vi "microstepping.vi"(4 "1 per 8 step":bool, 5 "1 per 16 step":bool, 6 "1 per 2 step":bool, 7 "full step":bool, 8 "1 per 4 step":bool, 9 "radius":dbl=5.0, 10 "arcLength":dbl=10.0, 11 "task/channels in microstepping":refnum<k21>) -> (0 "number of samples written":u32, 3 "convertedTodegree":dbl)   [LabVIEW 2016]
uses:
  <vilib>/DAQmx/write.llb/DAQmx Write (Digital 1D Bool NChan 1Samp 1Line).vi
  <vilib>/DAQmx/miscellaneous.llb/DAQmx Fill In Error Info.vi
panel:
  out "Numeric":i32
  out "full":dbl
  out "1 per 16":dbl
  in  "task/channels in trotate orientation":refnum<k21>="orientationPort2"
  in  "task/channels in toggle (step)":refnum<k21>="port01enable"
  in  "rotate orientation":string(combo)="clockwise"
  in  "steeper Motor Speed":u32(knob) scale=10.0..100.0
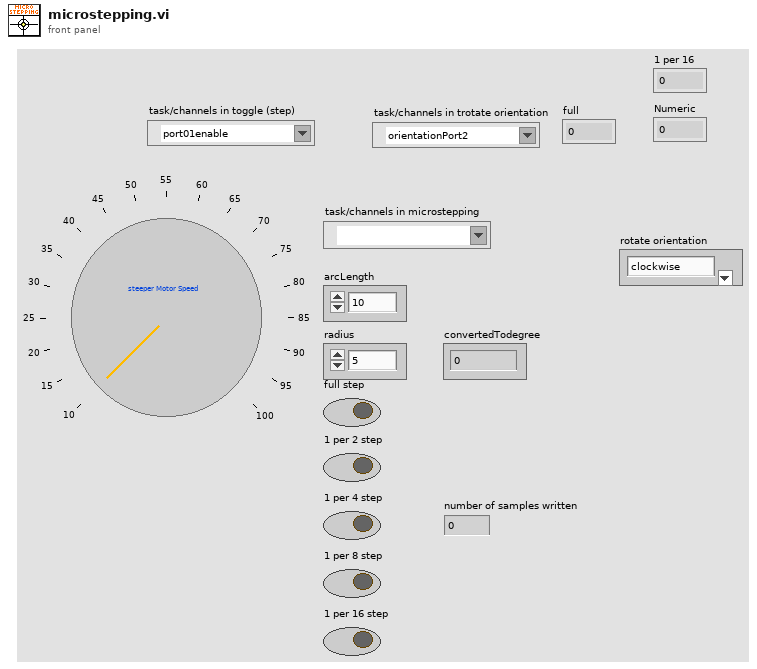
[diagram p1: front panel]
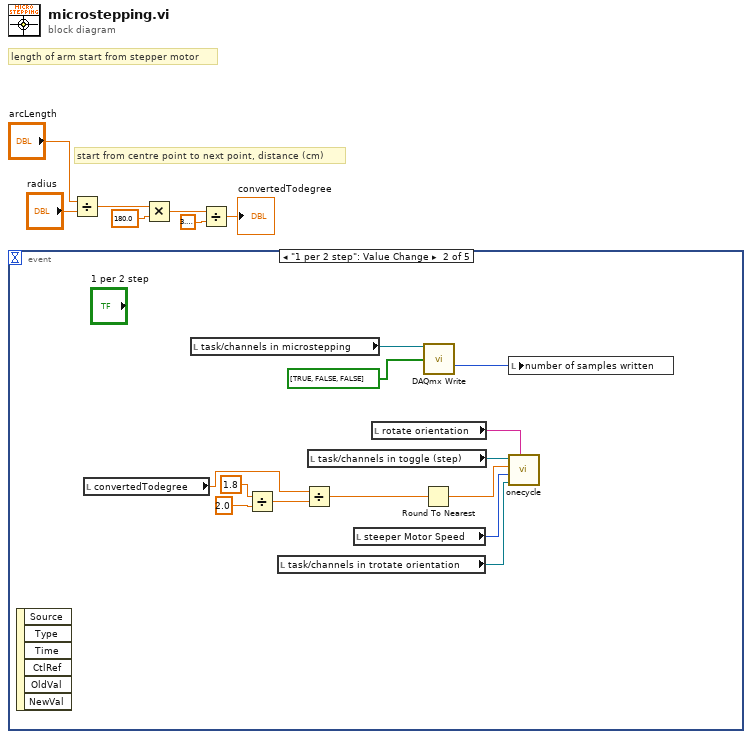
[diagram p0: block diagram]
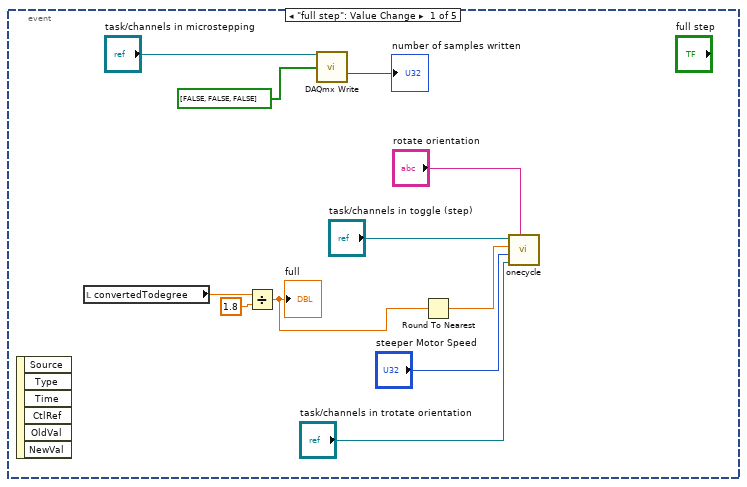
[diagram p2: hidden frame]
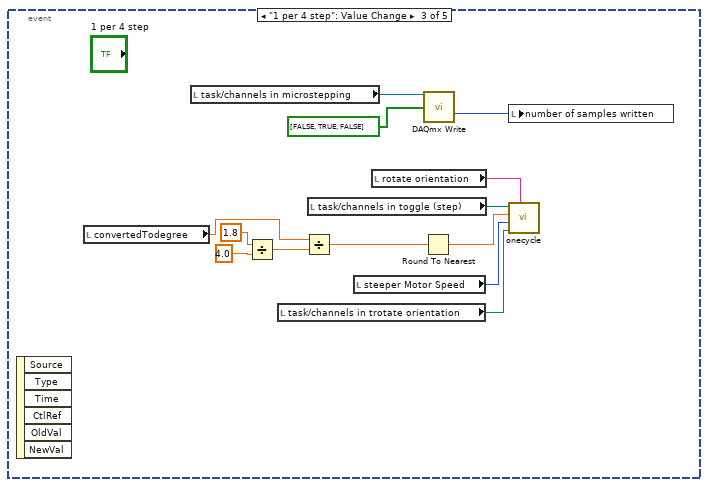
[diagram p3: hidden frame]
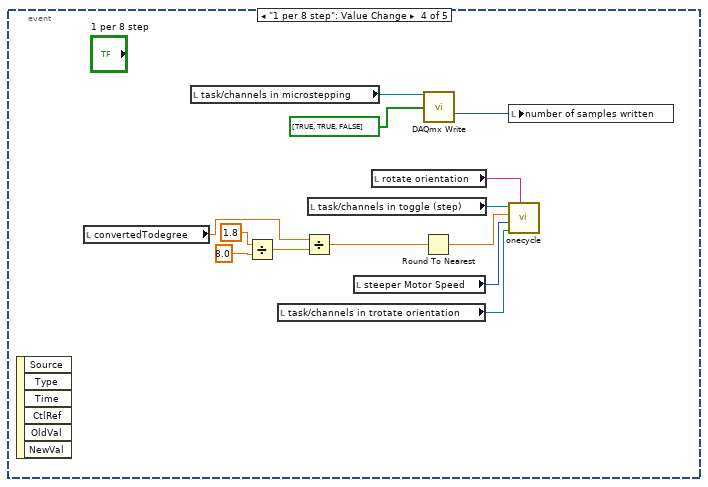
[diagram p4: hidden frame]
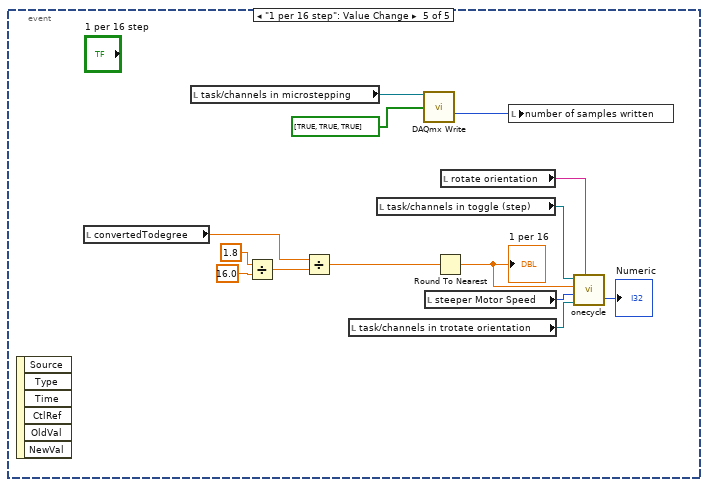
[diagram p5: hidden frame]
diagram:
  # "length of arm start from stepper motor"
  # "start from centre point to next point, distance (cm)"
  n1 = event shown="[1] \"1 per 2 step\": Value Change" {
    selector: _ -> [_ _ _ _ _]
    dyn-events: _ -> [_ _ _ _ _]
    timeout: _ -> [_ _ _ _ _]
    event "full step": Value Change {
      n2 = event-data() -> ()  [unwired: 1 in, 6 out]
      n3 = local read "convertedTodegree"() -> (w18:dbl)
      n4 = Divide(x=w18, y=1.8) -> (x/y=w9:dbl)
      "full" <- w9
      n5 = call-poly <vilib>:"DAQmx Write.vi"("task/channels in"="task/channels in microstepping", "data"=bool[] [FALSE, FALSE, FALSE]) -> ("number of samples written per channel"=→"number of samples written":u32)  [unwired: 11 in, 2 out]
      n6 = Round To Nearest(number=w9) -> (nearest integer value=w8:dbl)
      n7 = call "onecycle.vi"("rotate orientation"="rotate orientation", "task/channels in trotate orientation"="task/channels in trotate orientation", "steeper Motor Speed"="steeper Motor Speed", "no Of Step"=w8, "task/channels in toggle (step)"="task/channels in toggle (step)") -> ()  [unwired: 3 out]
    }
    event "1 per 2 step": Value Change {
      n8 = event-data() -> ()  [unwired: 1 in, 6 out]
      n9 = local read "convertedTodegree"() -> (w31:dbl)
      n10 = local read "task/channels in microstepping"() -> (w27:refnum<k21>)
      n11 = Divide(x=1.8 ("y"), y=2.0) -> (x/y=w28:dbl)
      n12 = local read "task/channels in trotate orientation"() -> (w22:refnum<k21>)
      n13 = Divide(x=w31, y=w28) -> (x/y=w24:dbl)
      n14 = local read "task/channels in toggle (step)"() -> (w20:refnum<k21>)
      n15 = local read "steeper Motor Speed"() -> (w21:u32)
      n16 = local read "rotate orientation"() -> (w23:string)
      n17 = Round To Nearest(number=w24) -> (nearest integer value=w19:dbl)
      n18 = call-poly <vilib>:"DAQmx Write.vi"("task/channels in"=w27, "data"=bool[] [TRUE, FALSE, FALSE]) -> ("number of samples written per channel"=w26:u32)  [unwired: 11 in, 2 out]
      n19 = local write "number of samples written"(w26) -> ()
      n20 = call "onecycle.vi"("rotate orientation"=w23, "task/channels in trotate orientation"=w22, "steeper Motor Speed"=w21, "no Of Step"=w19, "task/channels in toggle (step)"=w20) -> ()  [unwired: 3 out]
    }
    event "1 per 4 step": Value Change {
      n21 = event-data() -> ()  [unwired: 1 in, 6 out]
      n22 = local read "convertedTodegree"() -> (w41:dbl)
      n23 = local read "task/channels in microstepping"() -> (w39:refnum<k21>)
      n24 = Divide(x=1.8 ("y"), y=4.0) -> (x/y=w44:dbl)
      n25 = local read "task/channels in trotate orientation"() -> (w35:refnum<k21>)
      n26 = Divide(x=w41, y=w44) -> (x/y=w37:dbl)
      n27 = local read "task/channels in toggle (step)"() -> (w33:refnum<k21>)
      n28 = local read "steeper Motor Speed"() -> (w34:u32)
      n29 = local read "rotate orientation"() -> (w36:string)
      n30 = Round To Nearest(number=w37) -> (nearest integer value=w32:dbl)
      n31 = call-poly <vilib>:"DAQmx Write.vi"("task/channels in"=w39, "data"=bool[] [FALSE, TRUE, FALSE]) -> ("number of samples written per channel"=w38:u32)  [unwired: 11 in, 2 out]
      n32 = local write "number of samples written"(w38) -> ()
      n33 = call "onecycle.vi"("rotate orientation"=w36, "task/channels in trotate orientation"=w35, "steeper Motor Speed"=w34, "no Of Step"=w32, "task/channels in toggle (step)"=w33) -> ()  [unwired: 3 out]
    }
    event "1 per 8 step": Value Change {
      n34 = event-data() -> ()  [unwired: 1 in, 6 out]
      n35 = local read "convertedTodegree"() -> (w54:dbl)
      n36 = local read "task/channels in microstepping"() -> (w51:refnum<k21>)
      n37 = Divide(x=1.8 ("y"), y=8.0) -> (x/y=w55:dbl)
      n38 = local read "task/channels in trotate orientation"() -> (w47:refnum<k21>)
      n39 = Divide(x=w54, y=w55) -> (x/y=w50:dbl)
      n40 = local read "task/channels in toggle (step)"() -> (w46:refnum<k21>)
      n41 = local read "steeper Motor Speed"() -> (w48:u32)
      n42 = local read "rotate orientation"() -> (w49:string)
      n43 = Round To Nearest(number=w50) -> (nearest integer value=w45:dbl)
      n44 = call-poly <vilib>:"DAQmx Write.vi"("task/channels in"=w51, "data"=bool[] [TRUE, TRUE, FALSE]) -> ("number of samples written per channel"=w52:u32)  [unwired: 11 in, 2 out]
      n45 = local write "number of samples written"(w52) -> ()
      n46 = call "onecycle.vi"("rotate orientation"=w49, "task/channels in trotate orientation"=w47, "steeper Motor Speed"=w48, "no Of Step"=w45, "task/channels in toggle (step)"=w46) -> ()  [unwired: 3 out]
    }
    event "1 per 16 step": Value Change {
      n47 = event-data() -> ()  [unwired: 1 in, 6 out]
      n48 = local read "convertedTodegree"() -> (w69:dbl)
      n49 = local read "task/channels in microstepping"() -> (w66:refnum<k21>)
      n50 = Divide(x=1.8 ("y"), y=16.0) -> (x/y=w71:dbl)
      n51 = Divide(x=w69, y=w71) -> (x/y=w60:dbl)
      n52 = local read "task/channels in trotate orientation"() -> (w61:refnum<k21>)
      n53 = local read "task/channels in toggle (step)"() -> (w63:refnum<k21>)
      n54 = call-poly <vilib>:"DAQmx Write.vi"("task/channels in"=w66, "data"=bool[] [TRUE, TRUE, TRUE]) -> ("number of samples written per channel"=w65:u32)  [unwired: 11 in, 2 out]
      n55 = local read "steeper Motor Speed"() -> (w62:u32)
      n56 = Round To Nearest(number=w60) -> (nearest integer value=w58:dbl)
      "1 per 16" <- w58
      n57 = local read "rotate orientation"() -> (w64:string)
      n58 = local write "number of samples written"(w65) -> ()
      n59 = call "onecycle.vi"("rotate orientation"=w64, "task/channels in trotate orientation"=w61, "steeper Motor Speed"=w62, "no Of Step"=w58, "task/channels in toggle (step)"=w63) -> ("Numeric"=→"Numeric":i32)  [unwired: 2 out]
    }
  }
  n60 = Divide(x="arcLength", y="radius") -> (x/y=w1:dbl)
  n61 = Multiply(x=w1, y=180.0) -> (x*y=w3:dbl)
  n62 = Divide(x=w3, y=3.141592653589793) -> (x/y=→"convertedTodegree":dbl)
